vi "CLUSTER BASICS.vi"() -> ()   [LabVIEW 2018]
panel:
  out "Cluster 2":T1
  in  "Cluster":T1
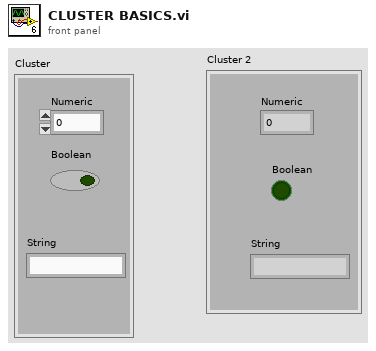
[diagram p1: front panel]
types:
  T1 = cluster{"Numeric":dbl, "Boolean":bool, "String":string}
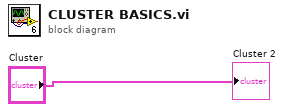
[diagram p0: block diagram]
diagram:
  "Cluster 2" <- "Cluster"
